vi "Simple_DAQ_AnalogIO.reset.vi"(0 "i ref in":refnum<vi>, 3 "Timeout":i32=10000, 5 "error in":errorcluster caption="Fehler (Eingang, kein Fehler)") -> (14 "i ref out":refnum<vi>, 17 "timed out":bool, 19 "error out":errorcluster caption="Fehler (Ausgang)")   [LabVIEW 2014, in "Simple_DAQ_AnalogIO.lvlib"]
doc: "Contact: Falk Ziegler, info@lab-coding.de"
uses:
  Simple_DAQ_AnalogIO.lvlib
  CSCore/CSApplicationBaseClasses/PSChannelBase/PSChannelBase.serviceType.ctl
  CSCore/CSApplicationBaseClasses/PSChannelBase/PSChannelBase.directionType.ctl
  CSlibraries/UtilityLib/UtilityLib.valueStatus.ctl
  <vilib>/DAQmx/write.llb/DAQmx Write (Analog DBL 1Chan 1Samp).vi
  CSlibraries/UtilityLib/UtilityLib.lvlib
  CSCore/CSApplicationBaseClasses/DeviceBase/DeviceBase.lvlib
  CSCore/CSApplicationBaseClasses/PSChannelBase/PSChannelBase.lvlib
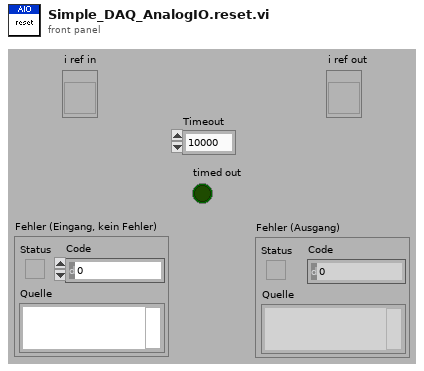
[diagram p1: front panel]
types:
  T1 = typedef "PSChannelBase.lvlib/PSChannelBase.directionType.ctl" = enum16{"unknown", "update actual value", "update nominal value", "update both"}
  T2 = typedef "PSChannelBase.lvlib/PSChannelBase.serviceType.ctl" = enum16{"onOff", "voltage", "current", "tripCurrent", "rampUpSpeed", "rampDownSpeed", "status"}
  T3 = typedef "UtilityLib.lvlib/UtilityLib.valueStatus.ctl" = enum16{"no info available", "stand by/off", "on", "warning", "alarm/malfunction", "not implemented", "user action required", "important information", "system default", "control default", "indicator default", "button default"}
  T4 = typedef "Simple_DAQ_AnalogIO.lvlib/Simple_DAQ_AnalogIO.i attribute.ctl" = cluster{"inputs":cluster{"index":i32[], "channel_task":refnum<k21>[], "range":cluster{"min":dbl, "max":dbl}[], "channel_number":i32, "scale_factor":dbl}, "outputs":cluster{"index":i32[], "channel_task":refnum<k21>[], "range":cluster{"min":dbl, "max":dbl}[], "channel_number":i32, "scale_factor":dbl}}
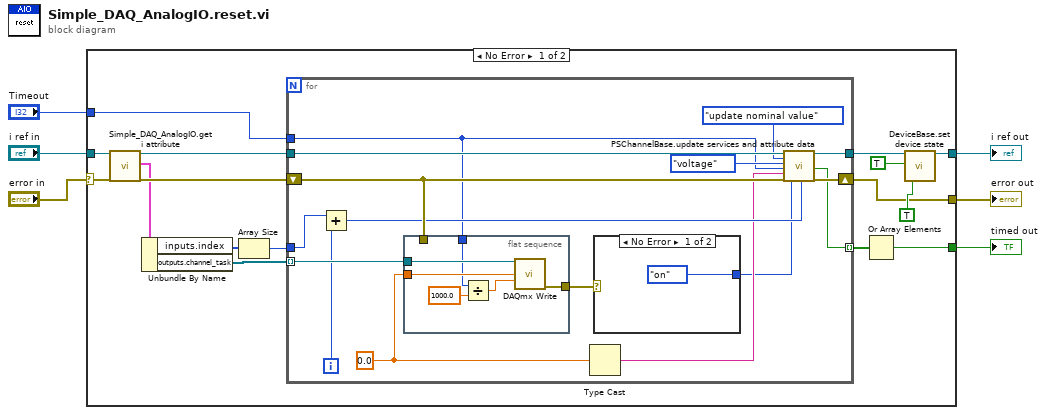
[diagram p0: block diagram]
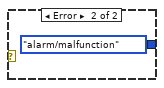
[diagram p2: hidden frame]
diagram:
  n1 = case shown="No Error" "error in" {
    selector: "error in" -> [w21 w47]
    tunnel: "i ref in" -> [w22 w48]
    tunnel: [w13 w48] -> w4
    tunnel: "Timeout" -> [w17 _]
    tunnel: [w14 _] -> w2
    tunnel: [w7 w47] -> w1
    frame No Error {
      n2 = call "Simple_DAQ_AnalogIO.get i attribute.vi"("i ref in"=w22, "error in (no error)"=w21) -> ("i ref out"=w20:refnum<vi>, "i attribute"=w18:T4, "error out"=w19:errorcluster)  [unwired: 15 in]
      n3 = Unbundle By Name(w18) -> ("inputs.index"=w9:i32[], "outputs.channel_task"=w16:refnum<k21>[])
      n4 = Array Size(array=w9) -> (size(s)=w8:i32)
      n5 = for {
        tunnel: w20 -> [w38]
        tunnel: w17 -> [w23]
        tunnel: [w36] -> w12
        tunnel: [w34] -> w15 mode=indexing
        tunnel: w16 -> [w28] mode=indexing
        shift-right: [w35] -> w7
        shift-left: w19 -> [w37]
        tunnel: w8 -> [w24]
        i -> [w25]
        w29 = 0.0
        n6 = Add(x=w24, y=w25) -> (x+y=w33:i32)
        n7 = flat-sequence {
          tunnel: w37 -> [_]
          tunnel: [w43] -> w31
          tunnel: w29 -> [w42]
          tunnel: w28 -> [w44]
          tunnel: w23 -> [w41]
          frame #0 {
            n8 = Divide(x=w41, y=1000.0) -> (x/y=w46:dbl)
            n9 = call-poly <vilib>:"DAQmx Write.vi"("task/channels in"=w44, "data"=w42, "timeout"=w46) -> ("error out"=w43:errorcluster)  [unwired: 10 in, 2 out]
          }
        }
        n10 = Type Cast(x=w29) -> (*(type *) &x=w32:string)  [unwired: 1 in]
        n11 = case shown="No Error" w31 {
          tunnel: [UtilityLib.valueStatus."on" ("quality") UtilityLib.valueStatus."alarm/malfunction" ("quality")] -> w30
          frame No Error {
          }
          frame Error {
          }
        }
        n12 = call "PSChannelBase.update services and attribute data.vi"("i ref in"=w38, "direction"=PSChannelBase.directionType."update nominal value", "service"=PSChannelBase.serviceType."voltage", "ms timeout (10000)"=w23, "value"=w32, "error in (no error)"=w37, "quality"=w30, "channelNumber"=w33) -> ("i ref out"=w36:refnum<vi>, "timed out"=w34:bool, "error out"=w35:errorcluster)  [unwired: 9 in]
      }
      n13 = Or Array Elements(Boolean array=w15) -> (logical OR=w14:bool)
      n14 = call "DeviceBase.set device state.vi"("i ref in"=w12, "implicit"=TRUE, "mayResetError (FALSE)"=TRUE) -> ("i ref out"=w13:refnum<vi>)  [unwired: 14 in, 2 out]
    }
    frame Error {
    }
  }
  "error out" <- w1
  "timed out" <- w2
  "i ref out" <- w4
